vi "GetFPOwner.vi"(6 "error in":errorcluster, 9 "GObj Refnum":refnum<vi>) -> (0 "error out":errorcluster, 3 "GObj Refnum out":refnum<vi>, 4 "owner UID":i32)   [LabVIEW 2014, in "Raspberry Pi Compatible Compiler for LabVIEW.lvlib" / "VI Interpreter.lvclass"]
uses:
  VI Interpreter.lvclass
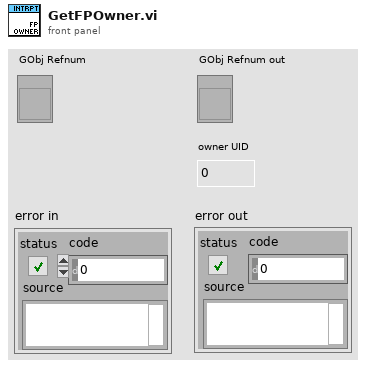
[diagram p1: front panel]
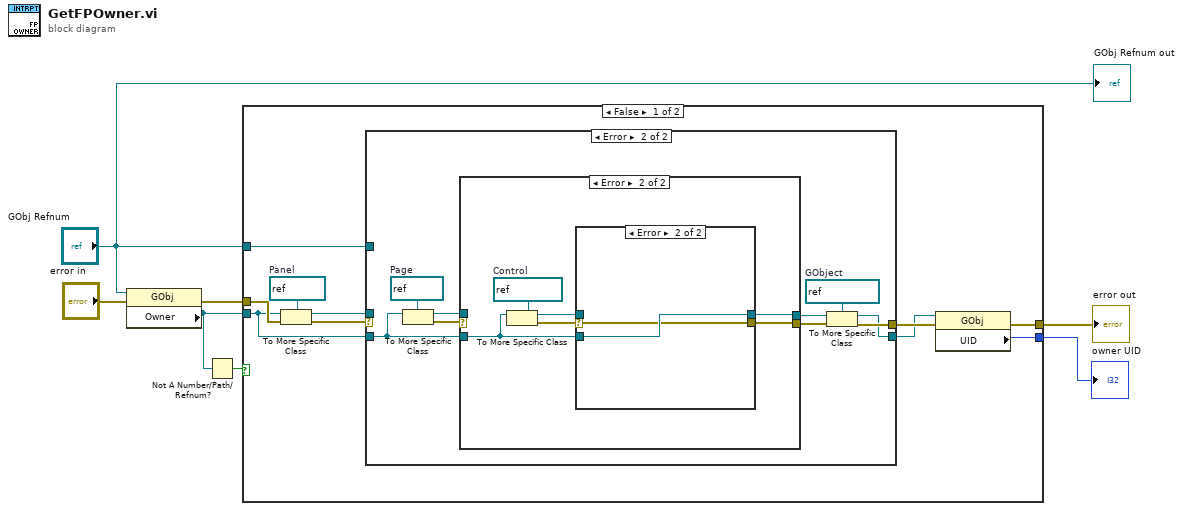
[diagram p0: block diagram]
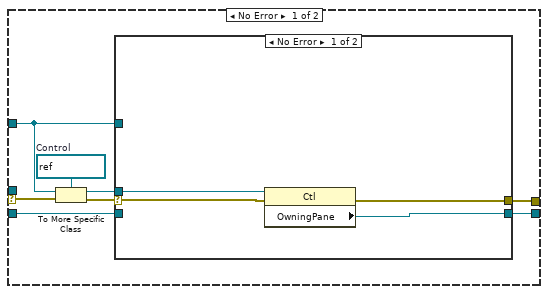
[diagram p2: hidden frame]
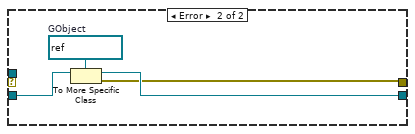
[diagram p3: hidden frame]
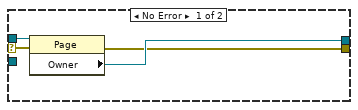
[diagram p4: hidden frame]
diagram:
  n1 = property class="GObj"(reference="GObj Refnum", error in="error in") -> (error out=w5:errorcluster, "Owner"=w3:refnum<vi>)  [unwired: 1 out]
  n2 = Not A Number/Path/Refnum?(number/path/refnum=w3) -> (NaN/Path/Refnum?=w2:bool)
  n3 = case shown="False" w2 {
    tunnel: [w12 _] -> w7
    tunnel: [w11 w57] -> w6
    tunnel: w5 -> [w10 w57]
    tunnel: "GObj Refnum" -> [w9 _]
    tunnel: w3 -> [w8 _]
    frame False {
      w17 = refnum<vi> refnum  # Panel
      n4 = To More Specific Class(target class=w17, reference=w8, error in=w10) -> (specific class reference=w16:refnum<vi>, error out=w15:errorcluster)
      n5 = case shown="Error" w15 {
        selector: w15 -> [w23 _]
        tunnel: w16 -> [_ _]
        tunnel: [w21 w40] -> w13
        tunnel: [w25 w41] -> w14
        tunnel: w9 -> [w19 _]
        tunnel: w8 -> [w18 w34]
        frame No Error {
          w24 = refnum<vi> refnum  # Control
          n6 = To More Specific Class(target class=w24, reference=w19, error in=w23) -> (specific class reference=w22:refnum<vi>, error out=w20:errorcluster)
          n7 = case shown="No Error" w20 {
            selector: w20 -> [w26 _]
            tunnel: [w29 w30] -> w25
            tunnel: w22 -> [w28 _]
            tunnel: [w27 w31] -> w21
            tunnel: w19 -> [_ _]
            tunnel: w18 -> [_ w32]
            frame No Error {
              n8 = property class="Ctl"(reference=w28, error in=w26) -> (error out=w29:errorcluster, "OwningPane"=w27:refnum<vi>)  [unwired: 1 out]
            }
            frame Error {
              w33 = refnum<vi> refnum  # GObject
              n9 = To More Specific Class(target class=w33, reference=w32) -> (specific class reference=w31:refnum<vi>, error out=w30:errorcluster)  [unwired: 1 in]
            }
          }
        }
        frame Error {
          w39 = refnum<vi> refnum  # Page
          w42 = refnum<vi> refnum  # GObject
          n10 = To More Specific Class(target class=w39, reference=w34) -> (specific class reference=w37:refnum<vi>, error out=w38:errorcluster)  [unwired: 1 in]
          n11 = case shown="Error" w38 {
            selector: w38 -> [w46 _]
            tunnel: w37 -> [w45 _]
            tunnel: [w44 w48] -> w36
            tunnel: [w43 w47] -> w35
            tunnel: w34 -> [_ w49]
            frame No Error {
              n12 = property class="Page"(reference=w45, error in=w46) -> (error out=w43:errorcluster, "Owner"=w44:refnum<vi>)  [unwired: 1 out]
            }
            frame Error {
              w52 = refnum<vi> refnum  # Control
              n13 = To More Specific Class(target class=w52, reference=w49) -> (specific class reference=w50:refnum<vi>, error out=w51:errorcluster)  [unwired: 1 in]
              n14 = case shown="Error" w51 {
                selector: w51 -> [w53 w55]
                tunnel: w50 -> [w54 _]
                tunnel: w49 -> [_ w56]
                tunnel: [w54 w56] -> w48
                tunnel: [w53 w55] -> w47
                frame No Error {
                }
                frame Error {
                }
              }
            }
          }
          n15 = To More Specific Class(target class=w42, reference=w36, error in=w35) -> (specific class reference=w40:refnum<vi>, error out=w41:errorcluster)
        }
      }
      n16 = property class="GObj"(reference=w13, error in=w14) -> (error out=w11:errorcluster, "UID"=w12:i32)  [unwired: 1 out]
    }
    frame True {
    }
  }
  "owner UID" <- w7
  "error out" <- w6
  "GObj Refnum out" <- "GObj Refnum"
